vi "Configure Alarm.vi"(0 "VISA resource name":refnum<visa-resource-name>, 1 "Source (0: Kelvin)":u16(ring) items=["Kelvin", "Celsius", "Sensor Units", "Linear Data"], 2 "High Value (0.0000)":dbl min=-99999.0 max=99999.0 step=0.0001 format="%.4f", 5 "Input (0: A)":u16(ring) items=["A", "B"], 7 "Alarm On/Off (F: Alarm OFF)":bool, 9 "Enable Latch  (F: OFF)":bool, 11 "error in (no error)":errorcluster, 12 "Low Value (0.0000)":dbl min=-100000.0 max=100000.0 step=0.0001 format="%.4f", 13 "Deadband (0.0000)":dbl min=-100000.0 max=100000.0 step=0.0001 format="%.4f") -> (4 "VISA resource name out":refnum<visa-resource-name>, 15 "error out":errorcluster)   [LabVIEW 2013, in "Lake Shore Cryotronics 331.lvlib"]
doc: "This VI configures the 331 alarm functions. Control is provided over the alarm high and low setpoints, trigger inside/outside status, audible alarm status, and alarm active status. A display annunciator and audible beeper signal an active alarm at the instrument."
uses:
  Lake Shore Cryotronics 331.lvlib
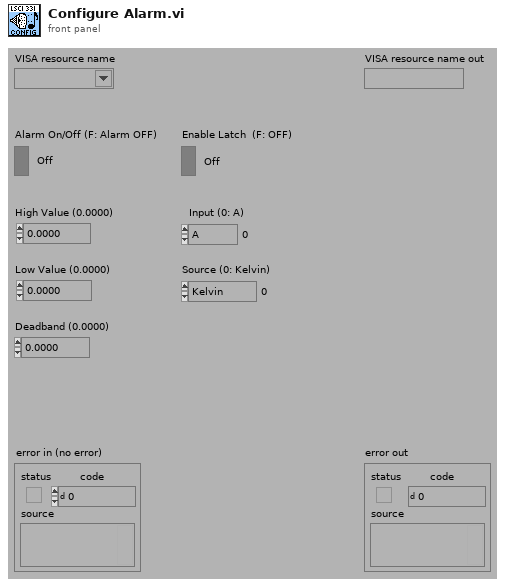
[diagram p1: front panel]
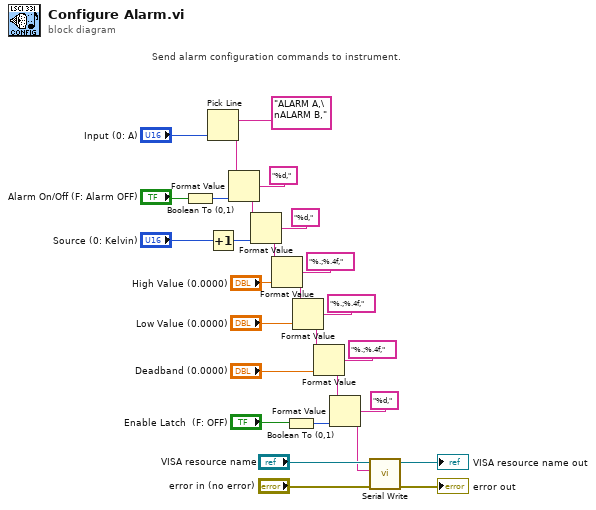
[diagram p0: block diagram]
diagram:
  # "Send alarm configuration commands to instrument."
  n1 = Boolean To (0,1)(Boolean="Alarm On/Off (F: Alarm OFF)") -> (0, 1=w20:i16)
  n2 = Pick Line(multi-line string="ALARM A,\nALARM B,", line index="Input (0: A)") -> (output string=w19:string)  [unwired: 1 in]
  n3 = Increment(x="Source (0: Kelvin)") -> (x+1=w16:u16)
  n4 = Format Value(string ("")=w19, format string="%d,", value (0)=w20) -> (output string=w15:string)
  n5 = Format Value(string ("")=w15, format string="%d,", value (0)=w16) -> (output string=w13:string)
  n6 = Format Value(string ("")=w13, format string="%.;%.4f,", value (0)="High Value (0.0000)") -> (output string=w10:string)
  n7 = Boolean To (0,1)(Boolean="Enable Latch  (F: OFF)") -> (0, 1=w8:i16)
  n8 = Format Value(string ("")=w10, format string="%.;%.4f,", value (0)="Low Value (0.0000)") -> (output string=w4:string)
  n9 = Format Value(string ("")=w4, format string="%.;%.4f,", value (0)="Deadband (0.0000)") -> (output string=w3:string)
  n10 = Format Value(string ("")=w3, format string="%d,", value (0)=w8) -> (output string=w2:string)
  n11 = call "Serial Write.vi"("error in (no error)"="error in (no error)", "Write Buffer (\"\")"=w2, "VISA resource name"="VISA resource name") -> ("error out"=→"error out":errorcluster, "VISA resource name out"=→"VISA resource name out":refnum<visa-resource-name>)  [unwired: 6 in, 1 out]
